vi "RoX_Tail_Interpolation.vi"() -> ()   [LabVIEW 2010]
doc: "In diesem Beispiel wird die Funktionsweise des VIs \"1D-Interpolation\" anhand von drei auswählbaren Testdatensätzen erläutert."
uses:
  <vilib>/gmath/NI_Gmath.lvlib
  CryoTUM_Mischer_Version_2-0/Instrument_Setup.vi
panel:
  in  "stop":bool caption="Stopp"
  in  "Method":i32(ring)=2 caption="Methode" items=["Nächste", "Linear", "Spline", "Hermite (kubisch)", "Lagrange"]
  # "Dieses Beispiel erläutert anhand von drei Testdatensätzen die Funktion des VIs \"1D-Interpolation\".\n\nAnweisungen:\n1) Führen Sie das VI aus.\n2) Wählen Sie Datensatz und Interpolationsmethode und beachten Sie die Resultate.\n3) Halten Sie das VI an. Weitere Informationen siehe Blockdiagramm."
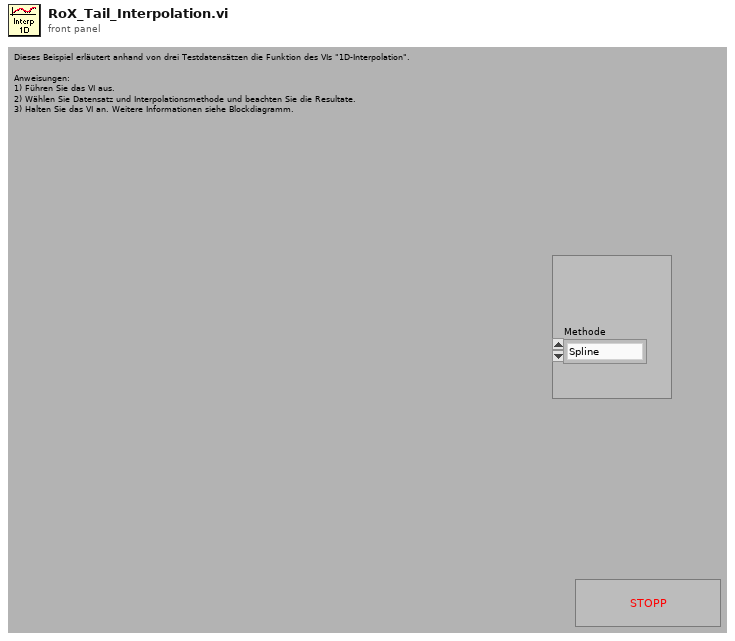
[diagram p1: front panel]
types:
  T1 = cluster{"starting value":dbl, "increment":dbl, "final value":dbl}
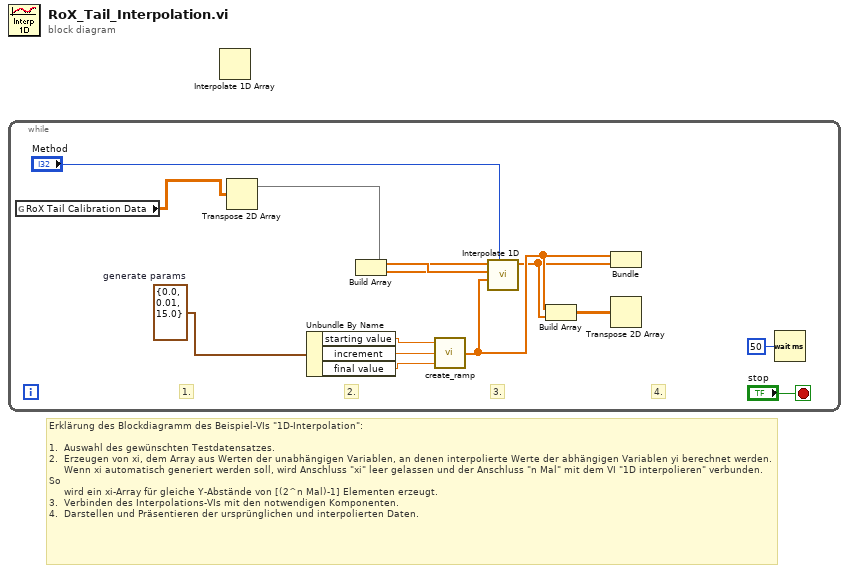
[diagram p0: block diagram]
diagram:
  # "Erklärung des Blockdiagramm des Beispiel-VIs \"1D-Interpolation\":\n\n1.  Auswahl des gewünschten Testdatensatzes.\n2.  Erzeugen von xi, dem Array aus Werten der unabhängigen Variablen, an denen interpolierte Werte der abhängigen Variablen yi berechnet werden. \n     Wenn xi automatisch generiert werden soll, wird Anschluss \"xi\" leer gelassen und der Anschluss \"n Mal\" mit dem VI \"1D interpolieren\" verbunden.  So\n     wird ein xi-Array für gleiche Y-Abstände von [(2^n Mal)-1] Elementen erzeugt.\n3.  Verbinden des Interpolations-VIs mit den notwendigen Komponenten.\n4.  Darstellen und Präsentieren der ursprünglichen und interpolierten Daten."
  n1 = while {
    stop <- "stop" stop-if-true
    w3 = T1 {"starting value"=0.0, "increment"=0.01, "final value"=15.0}  # generate params
    # "4."
    # "3."
    # "2."
    # "1."
    n2 = global read "Instrument_Setup.vi" "RoX Tail Calibration Data"() -> (w2:dbl[][])
    n3 = Transpose 2D Array(2D array=w2) -> (transposed array=w1:dbl[][])
    n4 = Unbundle By Name(w3) -> ("starting value"=w13:dbl, "increment"=w12:dbl, "final value"=w11:dbl)
    n5 = call "create_ramp.vi"("final value"=w11, "increment"=w12, "starting value"=w13) -> ("ramp data"=w7:dbl[])
    n6 = call <vilib>:"Interpolate 1D.vi"("method"="Method", "xi"=w7) -> ("yi"=w6:dbl[], "X"=w10:dbl[], "Y"=w9:dbl[])  [unwired: 5 in, 2 out]
    n7 = Build Array(w1, w10, w9) -> ()
    n8 = Build Array(w7, w6) -> (w8:dbl[][])
    n9 = Bundle("ramp data"=w7, "yi"=w6) -> ()  [unwired: 1 in, 1 out]
    n10 = Transpose 2D Array(2D array=w8) -> (transposed array=w5:dbl[][])
    n11 = Wait (ms)(milliseconds to wait=u32 50) -> ()  [unwired: 1 out]
  }
  n12 = Interpolate 1D Array() -> ()  [unwired: 2 in, 1 out]
